vi "ParamsHandlerTCP.vi"(7 "error":errorcluster, 9 "method":string, 10 "params_cluster":refnum<vi>[](array[refnum])) -> (0 "error":errorcluster, 3 "JSON-request":string)   [LabVIEW 2016]
panel:
  in  "api":i32=2
  in  "id":string="1"
  in  "jsonrpc":string="2.0"
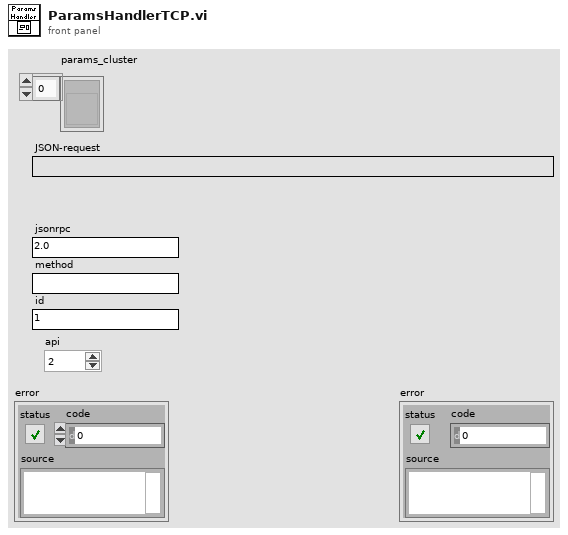
[diagram p1: front panel]
types:
  T1 = cluster{"jsonrpc":string, "method":string, "params":string[], "id":string, "api":i32}
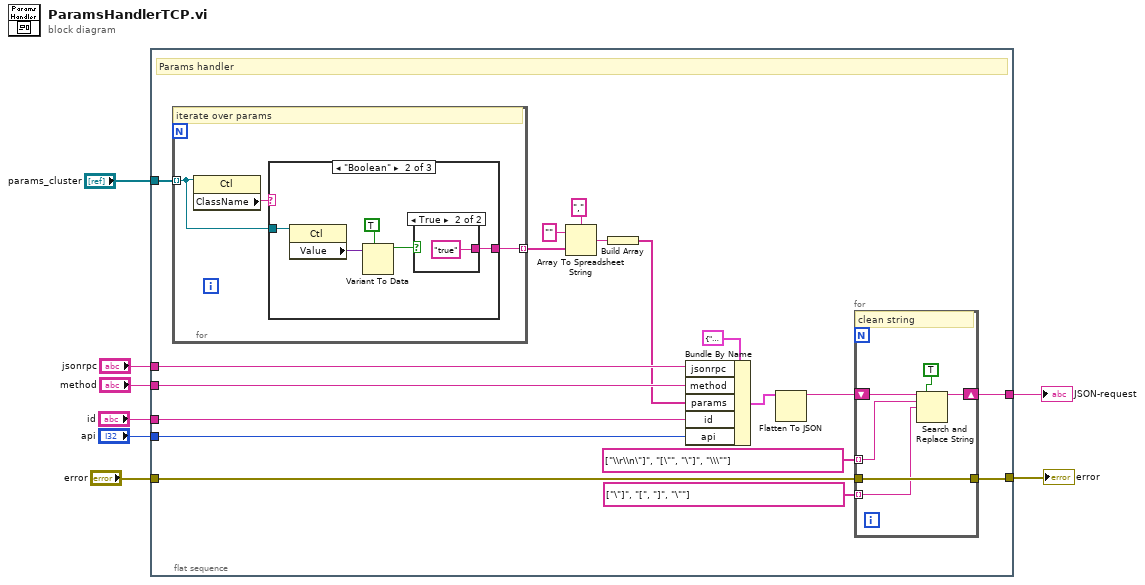
[diagram p0: block diagram]
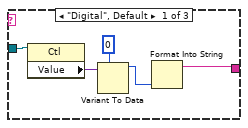
[diagram p2: hidden frame]
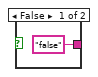
[diagram p3: hidden frame]
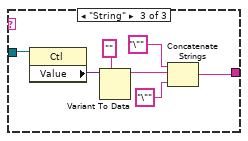
[diagram p4: hidden frame]
diagram:
  n1 = flat-sequence {
    tunnel: "error" -> [w16]
    tunnel: [w15] -> w7
    tunnel: "params_cluster" -> [w26]
    tunnel: "jsonrpc" -> [w23]
    tunnel: "method" -> [w22]
    tunnel: "id" -> [w21]
    tunnel: [w20] -> w2
    tunnel: "api" -> [w9]
    frame #0 {
      # "Params handler"
      n2 = for {
        tunnel: w26 -> [w34] mode=indexing
        tunnel: [w33] -> w14 mode=indexing
        # "iterate over params"
        n3 = property class="Ctl"(reference=w34) -> ("ClassName"=w35:string)  [unwired: 1 in, 2 out]
        n4 = case shown="\"Boolean\"" w35 {
          tunnel: w34 -> [w40 w45 w54]
          tunnel: [w36 w41 w50] -> w33
          frame "Digital", Default {
            n5 = property class="Ctl"(reference=w40) -> ("Value"=w38:variant)  [unwired: 1 in, 2 out]
            n6 = Variant To Data(type=0, Variant=w38) -> (data=w37:i32)  [unwired: 1 in, 1 out]
            n7 = Format Into String(w37) -> (resulting string=w36:string)  [unwired: 3 in, 1 out]
          }
          frame "Boolean" {
            n8 = property class="Ctl"(reference=w45) -> ("Value"=w43:variant)  [unwired: 1 in, 2 out]
            n9 = Variant To Data(type=TRUE, Variant=w43) -> (data=w42:bool)  [unwired: 1 in, 1 out]
            n10 = case shown="True" w42 {
              tunnel: ["false" "true"] -> w41
              frame False {
              }
              frame True {
              }
            }
          }
          frame "String" {
            n11 = property class="Ctl"(reference=w54) -> ("Value"=w53:variant)  [unwired: 1 in, 2 out]
            n12 = Variant To Data(type="", Variant=w53) -> (data=w51:string)  [unwired: 1 in, 1 out]
            n13 = Concatenate Strings("\"" ("string"), w51, "\"" ("string")) -> (w50:string)
          }
        }
      }
      n14 = Array To Spreadsheet String(delimiter (Tab)=",", array=w14, 3:"" ("format string")) -> (spreadsheet string=w11:string)
      n15 = Build Array(w11) -> (w10:string[])
      n16 = Bundle By Name(cluster=T1 {"jsonrpc"="", "method"="", "params"=[], "id"="", "api"=0} ("anything"), "jsonrpc"=w23, "method"=w22, "params"=w10, "id"=w21, "api"=w9) -> (w25:T1)
      n17 = Flatten To JSON(anything=w25) -> (JSON string=w19:string)  [unwired: 2 in, 1 out]
      n18 = for {
        tunnel: string[] ["\\r\\n\"]", "[\"", "\"]", "\\\""] ("search string") -> [w28] mode=indexing
        tunnel: string[] ["\"]", "[", "]", "\""] ("replace string (\"\")") -> [w27] mode=indexing
        shift-right: [w31] -> w20
        shift-left: w19 -> [w30]
        tunnel: w16 -> [w29]
        tunnel: [w29] -> w15
        # "clean string"
        n19 = Search and Replace String(replace all?=TRUE ("replace all? (F)"), input string=w30, search string=w28, replace string=w27) -> (result string=w31:string)  [unwired: 4 in, 3 out]
      }
    }
  }
  "error" <- w7
  "JSON-request" <- w2
